vi "Minicircuits rf power sensor read.vi"(6 "error in (no error)":errorcluster, 9 "Serial number (blank if only 1 unit)":string) -> (0 "error out":errorcluster, 3 "Power Read (dB)":dbl)   [LabVIEW 2013]
panel:
  in  "mcl_pm._USB_PM 2":refnum<k7>
  # "____________________________________________________________________________________________________"
  # "-  This is an example Of Mini-Circuits PWR-6g+ USB PowerMeter for 4 devices .\n-  The example use an acticeX , so before using this example make sure to install mcl_pm.dll \n-  To close the application , use the Stop Button . other wise disconnect and reconnect the Power meter to the USB port"
  # "Mini Circuits   PWR-6G+  Power Meter"
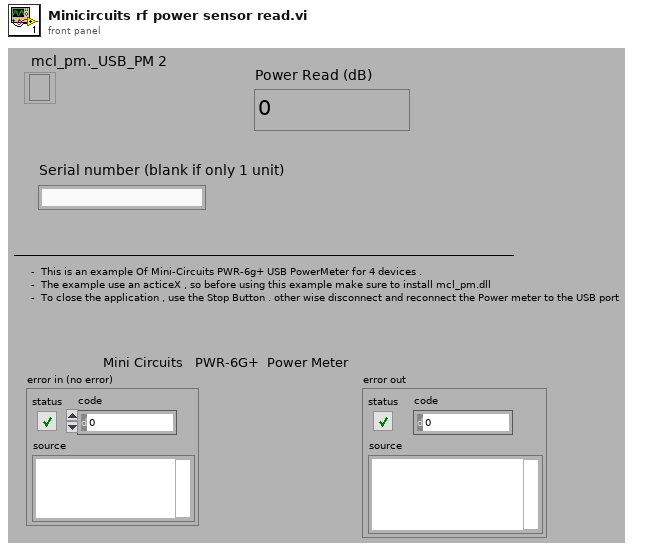
[diagram p1: front panel]
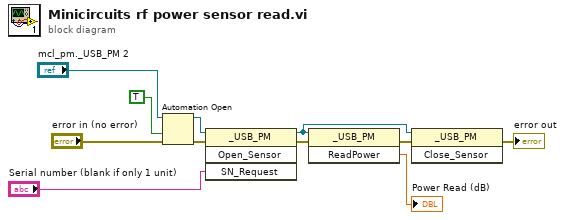
[diagram p0: block diagram]
diagram:
  n1 = Automation Open(error in (no error)="error in (no error)", Automation Refnum="mcl_pm._USB_PM 2", 9:TRUE ("open new instance (false)")) -> (Automation Refnum=w4:refnum<k7>, error out=w5:errorcluster)  [unwired: 1 in]
  n2 = invoke class="_USB_PM" method="Open_Sensor"(reference=w4, error in=w5, "SN_Request"="Serial number (blank if only 1 unit)") -> (reference out=w11:refnum<k7>, error out=w10:errorcluster)  [unwired: 1 in, 2 out]
  n3 = invoke class="_USB_PM" method="ReadPower"(reference=w11, error in=w10) -> (error out=w9:errorcluster, "ReadPower"=→"Power Read (dB)":sgl)  [unwired: 1 in, 1 out]
  n4 = invoke class="_USB_PM" method="Close_Sensor"(reference=w11, error in=w9) -> (error out=→"error out":errorcluster)  [unwired: 1 in, 2 out]
